vi "App Configuraton Extractor API.vi"(8 "error constant":errorcluster, 11 "App Cfg DVR":T1) -> (0 "error out":errorcluster, 3 "Application Configuration":T2)   [LabVIEW 2021, in "Configuration.lvlib"]
doc: "This method extracts is a Poliphormic method used to read each module configuration."
uses:
  Modules/Configuration/Configuration.lvlib
  Typedefs/Application Configuration.ctl
  Modules/Module Template/Typedefs/Config.ctl
  Modules/Core UI/Typedefs/Config.ctl
  Modules/Sound Manager/Typedefs/Config.ctl
  Modules/Configuration/Typedefs/App Cfg DVR.ctl
  Modules/Module Template/Module Template.lvlib
  Modules/Core UI/Board Game.lvlib
  Modules/Sound Manager/Sound Manager.lvlib
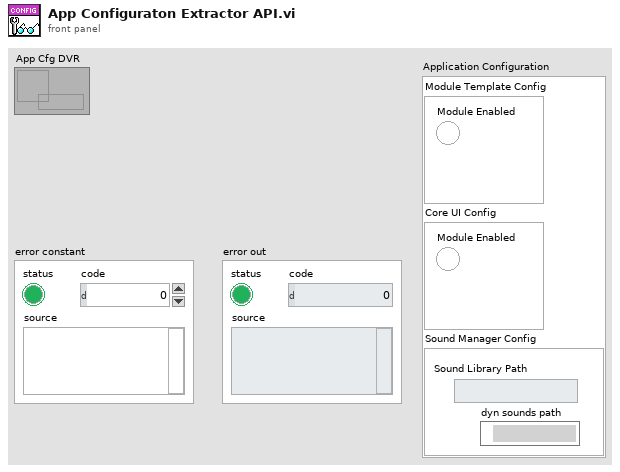
[diagram p1: front panel]
types:
  T1 = typedef "Configuration.lvlib/App Cfg DVR.ctl" = refnum<data-value>
  T2 = typedef "Configuration.lvlib/Application Configuration.ctl" = cluster{"Module Template Config":T3, "Core UI Config":T4, "Sound Manager Config":T5}
  T3 = typedef "Module Template.lvlib/Config.ctl" = cluster{"Module Enabled":bool}
  T4 = typedef "Board Game.lvlib/Config.ctl" = cluster{"Module Enabled":bool}
  T5 = typedef "Sound Manager.lvlib/Config.ctl" = cluster{"Sound Library Path":path, "dyn sounds path":path}
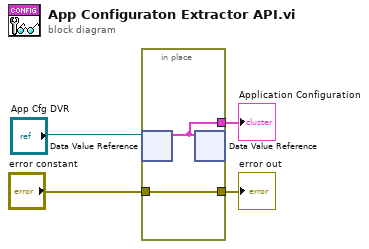
[diagram p0: block diagram]
diagram:
  n1 = in-place {
    in-place-border: [w6] -> w2
    in-place-border: "error constant" -> [w5]
    in-place-border: [w5] -> w3
    n2 = in-place-dvr #1("App Cfg DVR") -> (w6:T2)  [unwired: 1 out]
    n3 = in-place-dvr #1(w6) -> ()  [unwired: 2 out]
  }
  "error out" <- w3
  "Application Configuration" <- w2
